vi "Autonomous Independent.vi"() -> ()   [LabVIEW 2016]
doc: "This VI is called when autonomous begins, and will automatically be terminated when autonomous ends. You can carry out timed or sensor driven robot movement independently without needing to return to the caller."
uses:
  <vilib>/Rock Robotics/WPI/Solenoid/WPI_SolenoidValue.ctl
  <vilib>/Rock Robotics/WPI/SafetyOutput/WPI_SafetyOutputConfigMenu.ctl
  <vilib>/Rock Robotics/WPI/Utilities/WPI_GetSetVariantRefNum.vi
  <vilib>/Rock Robotics/Network Tables/NT Read String.vi
  <vilib>/Rock Robotics/Network Tables/NT Write Numeric Array.vi
  <vilib>/Rock Robotics/WPI/Ultrasonic/WPI_SonarMB1010AnalogRefNum Registry Get.vi
  <vilib>/Rock Robotics/WPI/RobotDrive/WPI_RobotDriveArcadeDrive_Standard(NoSaturation).vi
  <vilib>/Rock Robotics/WPI/Solenoid/WPI_SolenoidSetEnum.vi
  <vilib>/addons/control/pid/pid.llb/PID (DBL).vi
  <vilib>/Rock Robotics/WPI/Ultrasonic/WPI_SonarMB1010AnalogGetRange.vi
  <vilib>/Rock Robotics/WPI/ThirdParty/Sensors/ADIS16448 IMU/ADIS16448_IMU.lvlib
  <vilib>/addons/control/pid/NI_PID_pid.lvlib
panel:
  out "Current Movement, for debugging":T1 {"Y Joystick Value" scale=1.0..-1.0; "X Joystick Value" scale=-1.0..1.0}
  in  "Array of robot movements":T2(array[cluster])=[{"X Joystick Value"=0.39393939393939403, "Y Joystick Value"=0.0, "Delay (sec)"=1.0, "Movement Name"="turn"}, {"X Joystick Value"=-0.3737373737373737, "Y Joystick Value"=0.0, "Delay (sec)"=1.0, "Movement Name"="turn back"}] {"Y Joystick Value" scale=1.0..-1.0; "X Joystick Value" scale=-1.0..1.0}
  # "Be sure to right-click and choose Data Operations>>Make Current Value default if you want to save the array values with the VI"
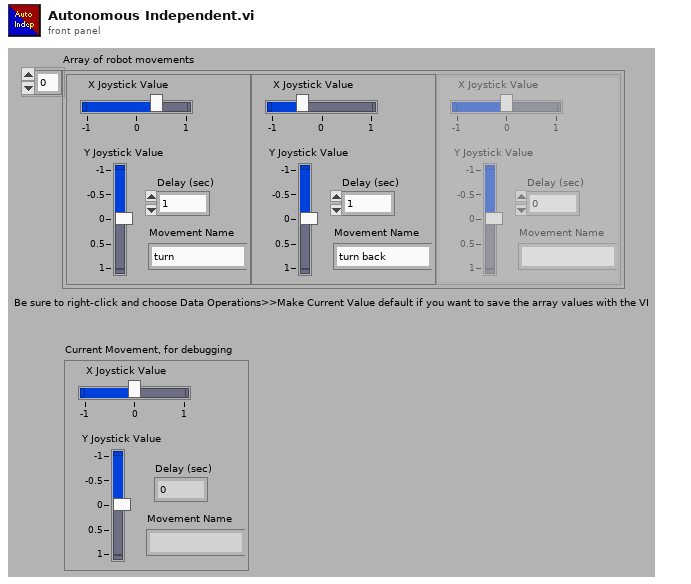
[diagram p1: front panel]
types:
  T1 = cluster{"X Joystick Value":dbl, "Y Joystick Value":dbl, "Delay (sec)":dbl, "Movement Name":string}
  T2 = cluster{"X Joystick Value":dbl, "Y Joystick Value":dbl, "Delay (sec)":dbl, "Movement Name":string}[]
  T3 = typedef "WPI_JoystickDevRef.ctl" = cluster{"Device":T4}
  T4 = typedef "WPI_JoystickDeviceEnum.ctl" = enum16{"USB 0", "USB 1", "USB 2", "USB 3", "USB 4", "USB 5"}
  T5 = typedef "WPI_RobotDriveDevRef.ctl" = cluster{"DevStatus":errorcluster, "Motors[]":T6[], "Square Inputs":bool, "Max Output":dbl}
  T6 = typedef "WPI_MotorControlDeviceRef.ctl" = cluster{"DeviceStatus":errorcluster, "Type":T7, "PWM":cluster{"PWM Channel":T8, "DeadBand":T9}, "CAN":cluster{"Device Number":u8, "SetOutput VI Ref":variant, "GetOutput VI Ref":variant, "Enable VI Ref":variant, "Disable VI Ref":variant, "Data":variant}, "Invert":bool}
  T7 = typedef "WPI_MotorControlType.ctl" = enum16{"PWM", "CAN"}
  T8 = typedef "FPGA_DIOPWMChannel.ctl" = enum8{"PWM 0", "PWM 1", "PWM 2", "PWM 3", "PWM 4", "PWM 5", "PWM 6", "PWM 7", "PWM 8", "PWM 9", "PWM MXP 0", "PWM MXP 1", "PWM MXP 2", "PWM MXP 3", "PWM MXP 4", "PWM MXP 5", "PWM MXP 6", "PWM MXP 7", "PWM MXP 8", "PWM MXP 9", "Invalid"}
  T9 = typedef "WPI_PWMDeadband.ctl" = cluster{"Name":string, "maxPositivePwm":i32, "minPositivePwm":i32, "centerPwm":i32, "maxNegativePwm":i32, "minNegativePwm":i32, "angularRange":u16}
  T10 = typedef "WPI_SonarMB1010AnalogDeviceRef.ctl" = cluster{"AIDeviceRef":T11, "Scaling factor (V/in)":dbl, "Average Bits":u8}
  T11 = typedef "WPI_AnalogChannelDevRef.ctl" = cluster{"DevStatus":errorcluster, "Analog Channel":T12}
  T12 = typedef "FPGA_AIChannel.ctl" = enum8{"AI 0", "AI 1", "AI 2", "AI 3", "AI MXP 0", "AI MXP 1", "AI MXP 2", "AI MXP 3", "Invalid"}
  T13 = typedef "WPI_SolenoidDevRef.ctl" = cluster{"DevStatus":errorcluster, "Pneumatics Control Module":u8, "Forward Solenoid Channel":T14, "Reverse Solenoid Channel":T14}
  T14 = typedef "WPI_SolenoidChannel.ctl" = enum8{"Solenoid 0", "Solenoid 1", "Solenoid 2", "Solenoid 3", "Solenoid 4", "Solenoid 5", "Solenoid 6", "Solenoid 7", "Invalid"}
  T15 = typedef "ADIS16448_IMU.lvlib/ADI_IMU_ADIS16448_InterruptDevRef.ctl" = cluster{"ADI IMU DevRef":T16, "InterruptRef":T18}
  T16 = typedef "ADIS16448_IMU.lvlib/ADI_IMU_ADIS16448_IMUDevRef.ctl" = cluster{"DevStatus":errorcluster, "Handle":i32, "SPI Bus":T17, "Device Found":bool, "Device Ready":bool, "Yaw Axis":enum16{"X", "Y", "Z"}, "AHRS Algorithm":enum16{"Complementary", "Madgwick"}, "Serial":u16, "Lot ID 2":u16, "Lot ID 1":u16, "Product ID":u16}
  T17 = typedef "spi_bus.ctl" = enum16{"SPI On-Board, CS0", "SPI On-Board, CS1", "SPI On-Board, CS2", "SPI On-Board, CS3", "SPI MXP", "Invalid"}
  T18 = typedef "WPI_InterruptRef.ctl" = cluster{"DevStatus":errorcluster, "InterruptIndex":T19}
  T19 = typedef "FPGA_InterruptIndex.ctl" = enum8{"0", "1", "2", "3", "4", "5", "6", "7", "Invalid"}
  T20 = typedef "WPI_SolenoidValue.ctl" = enum16{"Off", "On", "Forward", "Reverse"}
  T21 = typedef "WPI_SafetyOutputConfigMenu.ctl" = enum16{"Enable", "Disable"}
  T22 = cluster{"proportional gain (Kc)":dbl, "integral time (Ti, min)":dbl, "derivative time (Td, min)":dbl}
  T23 = cluster{"X Angle":dbl, "Y Angle":dbl, "Z Angle":dbl}
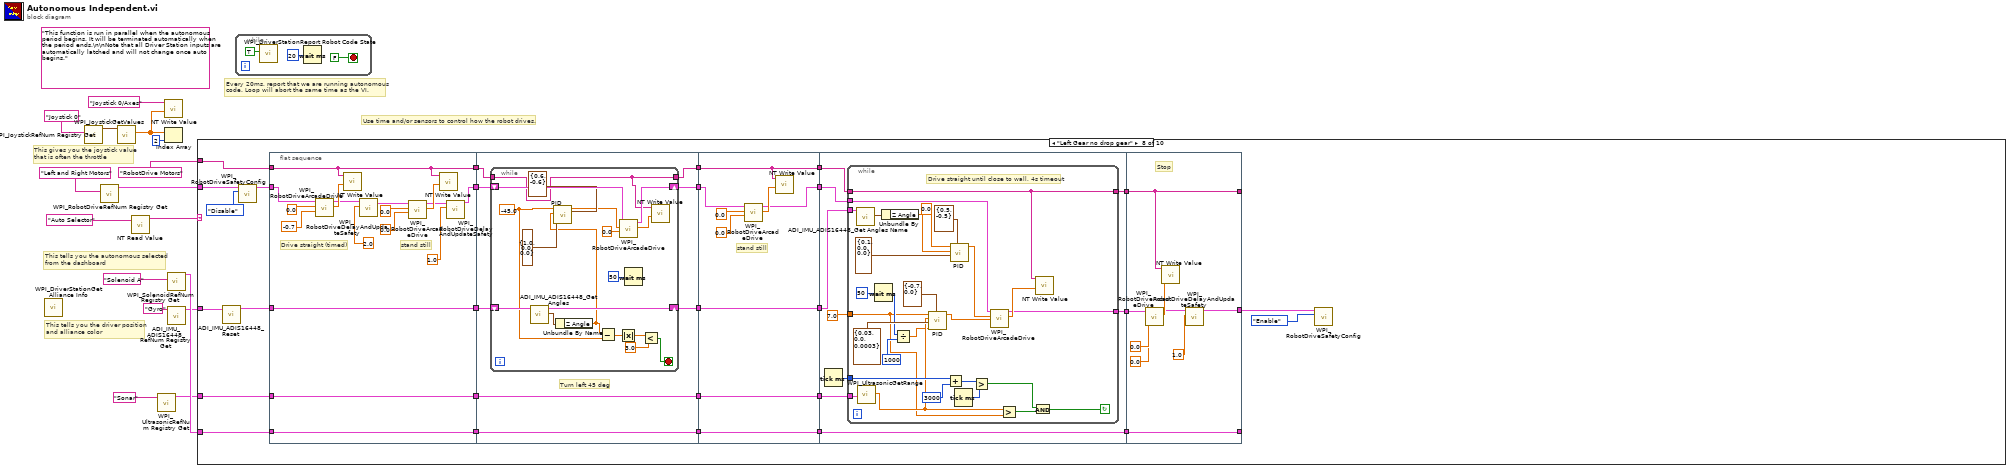
[diagram p0: block diagram]
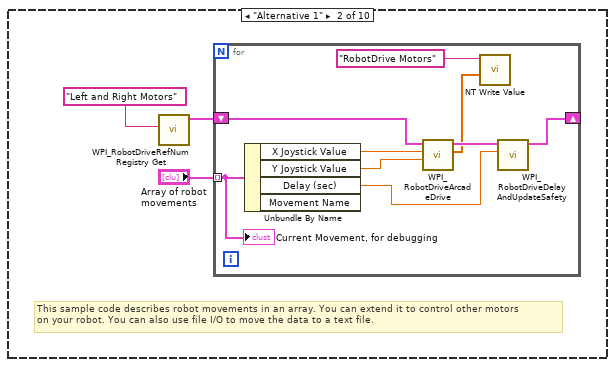
[diagram p3: hidden frame]
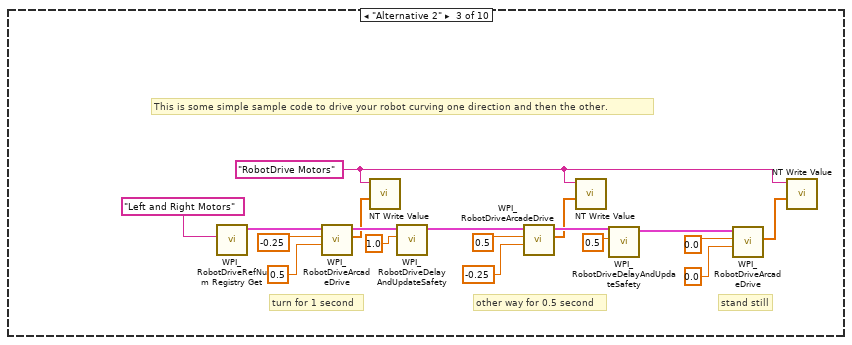
[diagram p4: hidden frame]
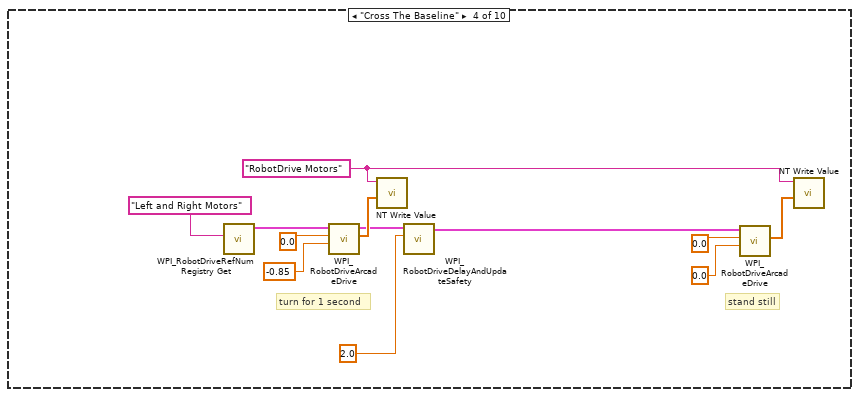
[diagram p5: hidden frame]
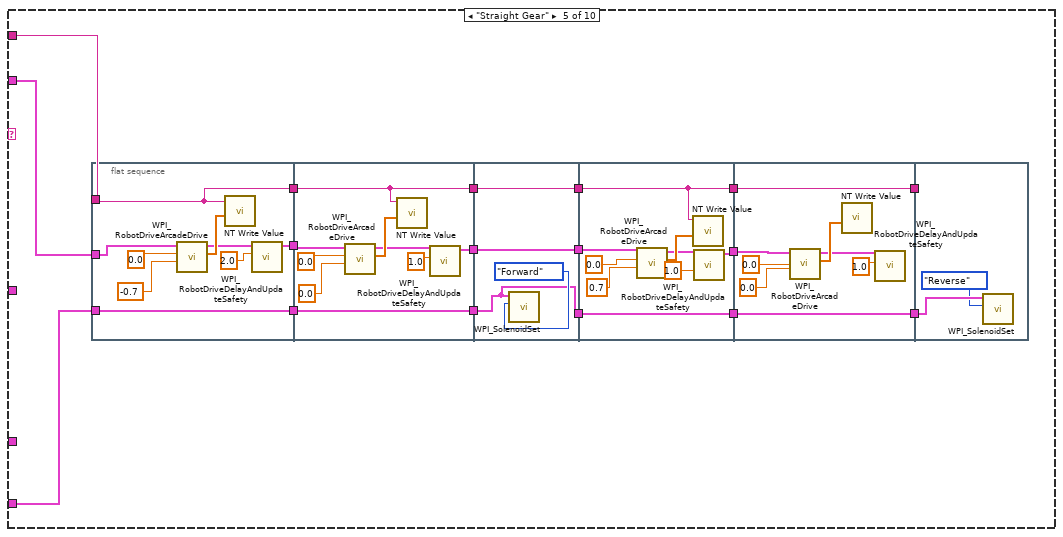
[diagram p6: hidden frame]
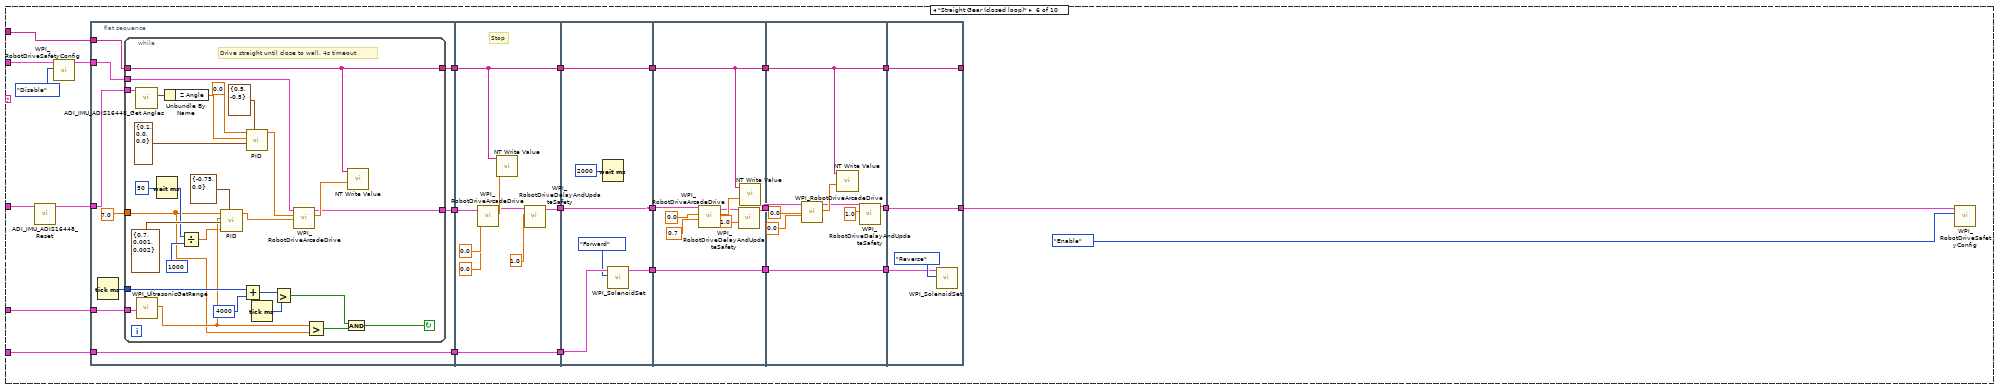
[diagram p7: hidden frame]
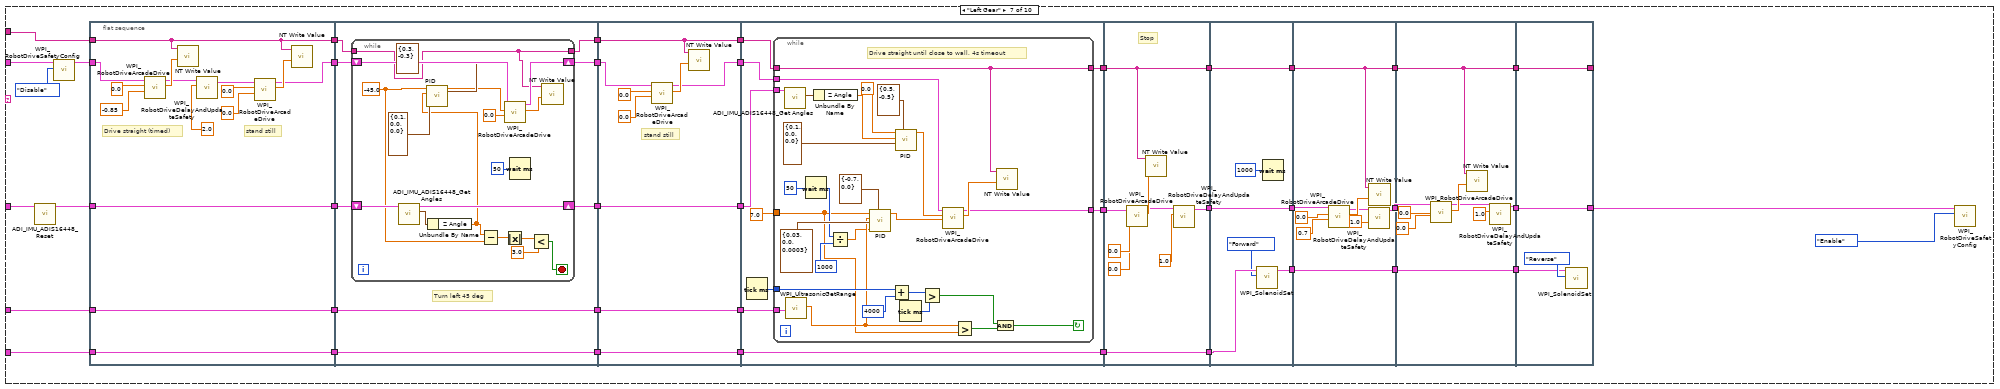
[diagram p8: hidden frame]
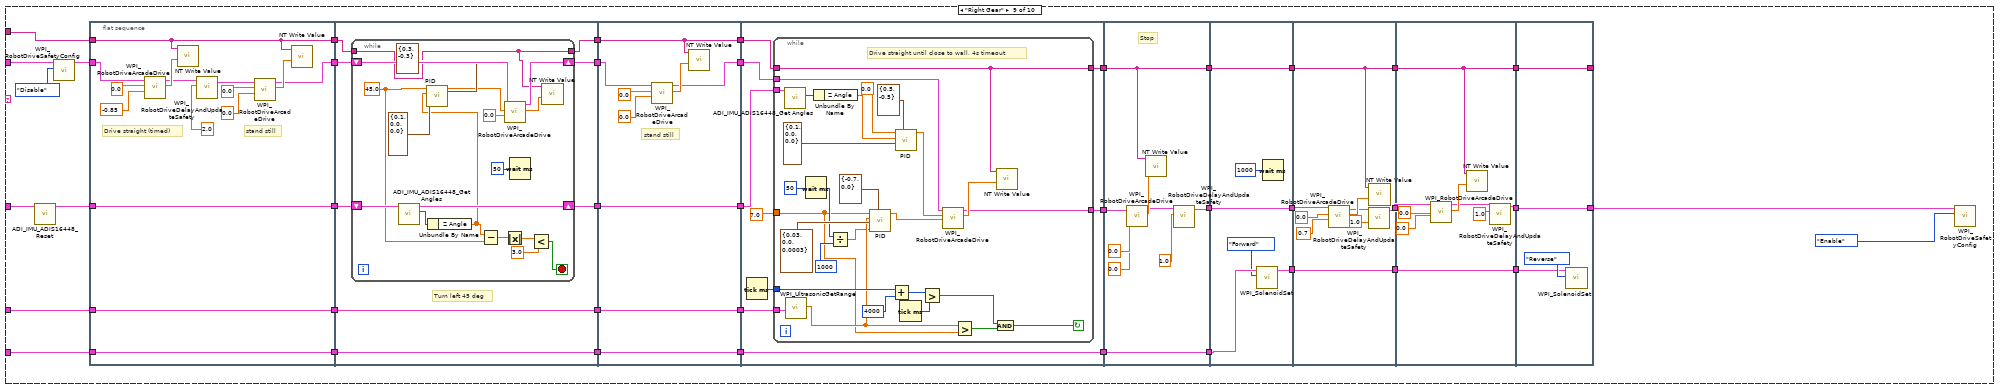
[diagram p9: hidden frame]
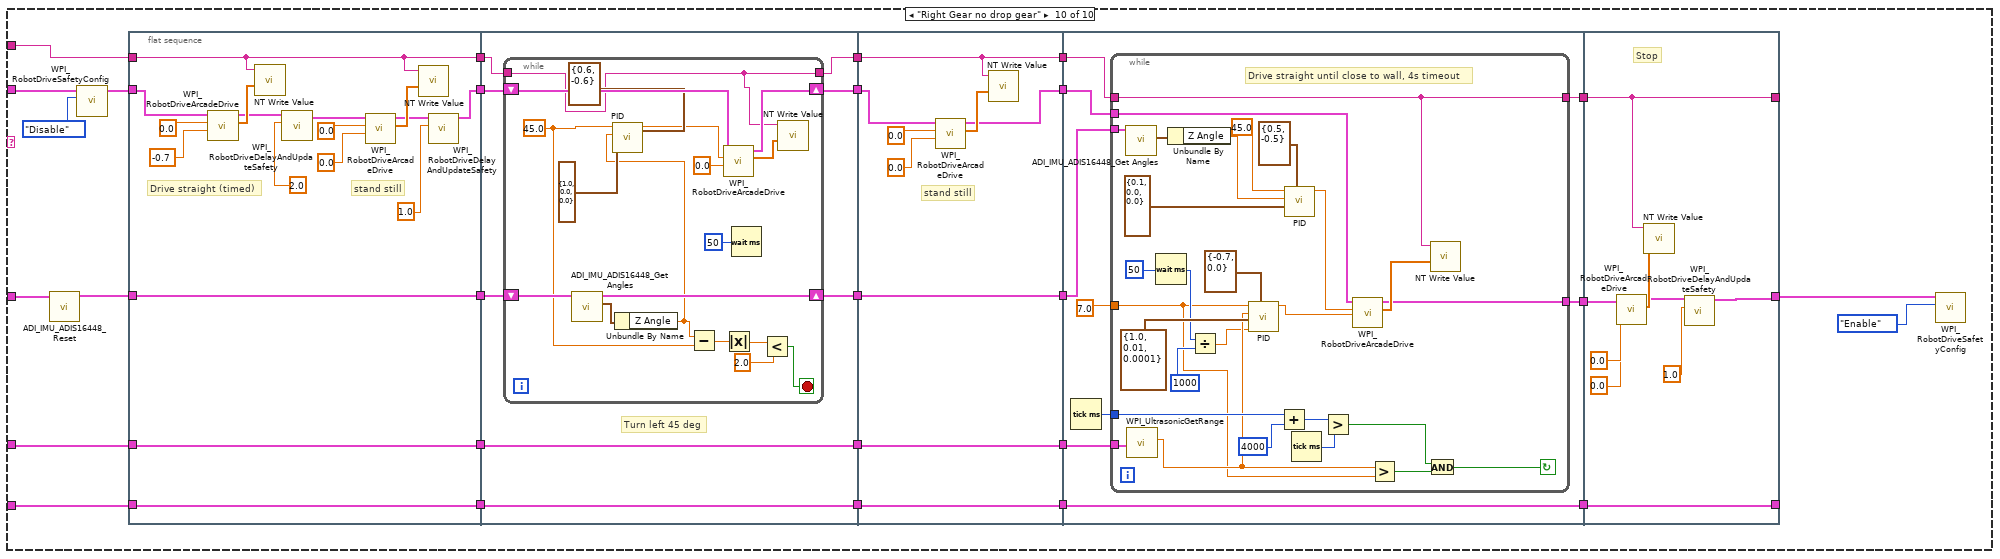
[diagram p10: hidden frame]
diagram:
  (unwired) "This function is run in parallel when the autonomous period begins. It will be terminated automatically when the period ends.\n\nNote that all Driver Station inputs are automatically latched and will not change once auto begins."
  # "This tells you the autonomous selected\nfrom the dashboard"
  # "Every 20ms, report that we are running autonomous\ncode. Loop will abort the same time as the VI."
  # "This gives you the joystick value\nthat is often the throttle"
  # "Use time and/or sensors to control how the robot drives."
  # "This tells you the driver position\nand alliance color"
  n1 = call <vilib>:"WPI_DriverStationGet Alliance Info.vi"() -> ()  [unwired: 12 out]
  n2 = call <vilib>:"WPI_JoystickRefNum Registry Get.vi"("refnum name"="Joystick 0") -> ("JoystickDevRef"=w15:T3)  [unwired: 1 in, 9 out]
  n3 = call <vilib>:"WPI_RobotDriveRefNum Registry Get.vi"("refnum name"="Left and Right Motors") -> ("RobotDriveDevRef"=w8:T5)  [unwired: 1 in, 9 out]
  n4 = call <vilib>:"WPI_JoystickGetValues.vi"("JoystickDevRef"=w15) -> ("Axes"=w11:dbl[])  [unwired: 6 in, 4 out]
  n5 = call-poly <vilib>:"NT Read Value.vi"("Name"="Auto Selector") -> ("String"=w12:string)  [unwired: 9 in, 1 out]
  n6 = call-poly <vilib>:"WPI_UltrasonicRefNum Registry Get.vi"("refnum name"="Sonar") -> ("SonarMB1010AnalogDevRef"=w1:T10)  [unwired: 9 in, 1 out]
  n7 = call-poly <vilib>:"NT Write Value.vi"("Numeric Array"=w11, "Name"="Joystick 0/Axes") -> ()  [unwired: 9 in, 1 out]
  n8 = Index Array(array=w11, index=2) -> ()  [unwired: 1 out]
  n9 = call <vilib>:"WPI_SolenoidRefNum Registry Get.vi"("refnum name"="Solenoid A") -> ("SolenoidDevRef"=w5:T13)  [unwired: 9 in, 1 out]
  n10 = call <vilib>:"ADI_IMU_ADIS16448_RefNum Registry Get.vi"("refnum name"="Gyro") -> ("ADI IMU Interrupt DevRef"=w3:T15)  [unwired: 9 in, 1 out]
  n11 = case shown="\"Left Gear no drop gear\"" w12 {
    tunnel: w8 -> [_ _ _ _ w75 w136 w249 w400 w537 w688]
    tunnel: "RobotDrive Motors" ("Name") -> [_ _ _ _ w74 w138 w251 w402 w539 w690]
    tunnel: w5 -> [_ _ _ _ w69 w137 w250 w401 w538 w689]
    tunnel: w3 -> [_ _ _ _ _ w141 w254 w405 w542 w693]
    tunnel: w1 -> [_ _ _ _ _ w140 w253 w404 w541 w692]
    frame Default {
      # "You can put your main auto here, or you can right-click on the case and make any\nother frame be the default case."
      # "This is the frame that will execute if no selection is made, or if it is not recognized"
    }
    frame "Alternative 1" {
      # "This sample code describes robot movements in an array. You can extend it to control other motors\non your robot. You can also use file I/O to move the data to a text file."
      n12 = call <vilib>:"WPI_RobotDriveRefNum Registry Get.vi"("refnum name"="Left and Right Motors") -> ("RobotDriveDevRef"=w18:T5)  [unwired: 1 in, 9 out]
      n13 = for {
        shift-right: [w26] -> _
        shift-left: w18 -> [w27]
        tunnel: "Array of robot movements" -> [w22] mode=indexing
        n14 = Unbundle By Name(w22) -> ("X Joystick Value"=w25:dbl, "Y Joystick Value"=w24:dbl, "Delay (sec)"=w23:dbl)  [unwired: 1 out]
        n15 = call-poly <vilib>:"WPI_RobotDriveArcadeDrive.vi"("Y axis value"=w24, "X axis value"=w25, "RobotDriveDevRef"=w27) -> ("Motor Values"=w20:dbl[], "RobotDriveDevRef"=w28:T5)  [unwired: 1 in, 6 out]
        n16 = call-poly <vilib>:"NT Write Value.vi"("Numeric Array"=w20, "Name"="RobotDrive Motors") -> ()  [unwired: 9 in, 1 out]
        n17 = call <vilib>:"WPI_RobotDriveDelayAndUpdateSafety.vi"("Delay (s)"=w23, "RobotDriveDevRef"=w28) -> ("RobotDriveDevRef 2"=w26:T5)  [unwired: 8 in, 1 out]
        "Current Movement, for debugging" <- w22
      }
    }
    frame "Alternative 2" {
      w30 = "RobotDrive Motors" ("Name")
      # "This is some simple sample code to drive your robot curving one direction and then the other."
      # "stand still"
      # "other way for 0.5 second"
      # "turn for 1 second"
      n18 = call <vilib>:"WPI_RobotDriveRefNum Registry Get.vi"("refnum name"="Left and Right Motors") -> ("RobotDriveDevRef"=w46:T5)  [unwired: 1 in, 9 out]
      n19 = call-poly <vilib>:"WPI_RobotDriveArcadeDrive.vi"("Y axis value"=0.5 ("X axis value"), "X axis value"=-0.25, "RobotDriveDevRef"=w46) -> ("Motor Values"=w29:dbl[], "RobotDriveDevRef"=w39:T5)  [unwired: 1 in, 6 out]
      n20 = call-poly <vilib>:"NT Write Value.vi"("Numeric Array"=w29, "Name"=w30) -> ()  [unwired: 9 in, 1 out]
      n21 = call <vilib>:"WPI_RobotDriveDelayAndUpdateSafety.vi"("Delay (s)"=1.0, "RobotDriveDevRef"=w39) -> ("RobotDriveDevRef 2"=w40:T5)  [unwired: 8 in, 1 out]
      n22 = call-poly <vilib>:"WPI_RobotDriveArcadeDrive.vi"("Y axis value"=-0.25 ("X axis value"), "X axis value"=0.5, "RobotDriveDevRef"=w40) -> ("Motor Values"=w31:dbl[], "RobotDriveDevRef"=w41:T5)  [unwired: 1 in, 6 out]
      n23 = call-poly <vilib>:"NT Write Value.vi"("Numeric Array"=w31, "Name"=w30) -> ()  [unwired: 9 in, 1 out]
      n24 = call <vilib>:"WPI_RobotDriveDelayAndUpdateSafety.vi"("Delay (s)"=0.5, "RobotDriveDevRef"=w41) -> ("RobotDriveDevRef 2"=w42:T5)  [unwired: 8 in, 1 out]
      n25 = call-poly <vilib>:"WPI_RobotDriveArcadeDrive.vi"("Y axis value"=0.0 ("X axis value"), "X axis value"=0.0, "RobotDriveDevRef"=w42) -> ("Motor Values"=w32:dbl[])  [unwired: 1 in, 7 out]
      n26 = call-poly <vilib>:"NT Write Value.vi"("Numeric Array"=w32, "Name"=w30) -> ()  [unwired: 9 in, 1 out]
    }
    frame "Cross The Baseline" {
      w57 = "RobotDrive Motors" ("Name")
      # "stand still"
      # "turn for 1 second"
      n27 = call <vilib>:"WPI_RobotDriveRefNum Registry Get.vi"("refnum name"="Left and Right Motors") -> ("RobotDriveDevRef"=w48:T5)  [unwired: 1 in, 9 out]
      n28 = call-poly <vilib>:"WPI_RobotDriveArcadeDrive.vi"("Y axis value"=-0.85 ("X axis value"), "X axis value"=0.0, "RobotDriveDevRef"=w48) -> ("Motor Values"=w58:dbl[], "RobotDriveDevRef"=w51:T5)  [unwired: 1 in, 6 out]
      n29 = call-poly <vilib>:"NT Write Value.vi"("Numeric Array"=w58, "Name"=w57) -> ()  [unwired: 9 in, 1 out]
      n30 = call <vilib>:"WPI_RobotDriveDelayAndUpdateSafety.vi"("Delay (s)"=2.0, "RobotDriveDevRef"=w51) -> ("RobotDriveDevRef 2"=w47:T5)  [unwired: 8 in, 1 out]
      n31 = call-poly <vilib>:"WPI_RobotDriveArcadeDrive.vi"("Y axis value"=0.0 ("X axis value"), "X axis value"=0.0, "RobotDriveDevRef"=w47) -> ("Motor Values"=w56:dbl[])  [unwired: 1 in, 7 out]
      n32 = call-poly <vilib>:"NT Write Value.vi"("Numeric Array"=w56, "Name"=w57) -> ()  [unwired: 9 in, 1 out]
    }
    frame "Straight Gear" {
      n33 = flat-sequence {
        tunnel: w75 -> [w79]
        tunnel: w74 -> [w77]
        tunnel: [w78] -> w73
        tunnel: [w77] -> w72
        tunnel: w69 -> [w76]
        tunnel: [w76] -> w68
        tunnel: w73 -> [w88]
        tunnel: w72 -> [w87]
        tunnel: [w87] -> w71
        tunnel: w68 -> [w86]
        tunnel: [w86] -> w67
        tunnel: [w85] -> w64
        tunnel: w71 -> [w97]
        tunnel: [w97] -> w70
        tunnel: w67 -> [w94]
        tunnel: w64 -> [w95]
        tunnel: [w95] -> w63
        tunnel: [w94] -> w61
        tunnel: w70 -> [w103]
        tunnel: [w103] -> w66
        tunnel: w63 -> [w102]
        tunnel: [w99] -> w62
        tunnel: w61 -> [w101]
        tunnel: [w101] -> w60
        tunnel: w66 -> [w114]
        tunnel: [w114] -> w65
        tunnel: w62 -> [w108]
        tunnel: w60 -> [w107]
        tunnel: [w107] -> w59
        tunnel: w65 -> [_]
        tunnel: w59 -> [w116]
        frame #0 {
          n34 = call-poly <vilib>:"WPI_RobotDriveArcadeDrive.vi"("Y axis value"=-0.7 ("X axis value"), "X axis value"=0.0, "RobotDriveDevRef"=w79) -> ("Motor Values"=w84:dbl[], "RobotDriveDevRef"=w81:T5)  [unwired: 1 in, 6 out]
          n35 = call-poly <vilib>:"NT Write Value.vi"("Numeric Array"=w84, "Name"=w77) -> ()  [unwired: 9 in, 1 out]
          n36 = call <vilib>:"WPI_RobotDriveDelayAndUpdateSafety.vi"("Delay (s)"=2.0, "RobotDriveDevRef"=w81) -> ("RobotDriveDevRef 2"=w78:T5)  [unwired: 8 in, 1 out]
        }
        frame #1 {
          n37 = call-poly <vilib>:"WPI_RobotDriveArcadeDrive.vi"("Y axis value"=0.0 ("X axis value"), "X axis value"=0.0, "RobotDriveDevRef"=w88) -> ("Motor Values"=w93:dbl[], "RobotDriveDevRef"=w90:T5)  [unwired: 1 in, 6 out]
          n38 = call-poly <vilib>:"NT Write Value.vi"("Numeric Array"=w93, "Name"=w87) -> ()  [unwired: 9 in, 1 out]
          n39 = call <vilib>:"WPI_RobotDriveDelayAndUpdateSafety.vi"("Delay (s)"=1.0, "RobotDriveDevRef"=w90) -> ("RobotDriveDevRef 2"=w85:T5)  [unwired: 8 in, 1 out]
        }
        frame #2 {
          n40 = call-poly <vilib>:"WPI_SolenoidSet.vi"("Value"=WPI_SolenoidValue."Forward", "SolenoidDevRef"=w94) -> ()  [unwired: 8 in, 2 out]
        }
        frame #3 {
          w98 = 1.0 ("Delay (s)")
          n41 = call-poly <vilib>:"WPI_RobotDriveArcadeDrive.vi"("Y axis value"=0.7 ("X axis value"), "X axis value"=0.0, "RobotDriveDevRef"=w102) -> ("Motor Values"=w106:dbl[], "RobotDriveDevRef"=w100:T5)  [unwired: 1 in, 6 out]
          n42 = call-poly <vilib>:"NT Write Value.vi"("Numeric Array"=w106, "Name"=w103) -> ()  [unwired: 9 in, 1 out]
          n43 = call <vilib>:"WPI_RobotDriveDelayAndUpdateSafety.vi"("Feed time (s)"=w98, "Delay (s)"=w98, "RobotDriveDevRef"=w100) -> ("RobotDriveDevRef 2"=w99:T5)  [unwired: 7 in, 1 out]
        }
        frame #4 {
          n44 = call-poly <vilib>:"WPI_RobotDriveArcadeDrive.vi"("Y axis value"=0.0 ("X axis value"), "X axis value"=0.0, "RobotDriveDevRef"=w108) -> ("Motor Values"=w113:dbl[], "RobotDriveDevRef"=w111:T5)  [unwired: 1 in, 6 out]
          n45 = call-poly <vilib>:"NT Write Value.vi"("Numeric Array"=w113) -> ()  [unwired: 10 in, 1 out]
          n46 = call <vilib>:"WPI_RobotDriveDelayAndUpdateSafety.vi"("Delay (s)"=1.0, "RobotDriveDevRef"=w111) -> ()  [unwired: 8 in, 2 out]
        }
        frame #5 {
          n47 = call-poly <vilib>:"WPI_SolenoidSet.vi"("Value"=WPI_SolenoidValue."Reverse", "SolenoidDevRef"=w116) -> ()  [unwired: 8 in, 2 out]
        }
      }
    }
    frame "Straight Gear (closed loop)" {
      n48 = call <vilib>:"ADI_IMU_ADIS16448_Reset.vi"("ADI IMU Interrupt DevRef"=w141) -> ("ADI IMU Interrupt DevRef Out"=w139:T15)  [unwired: 9 in, 1 out]
      n49 = call <vilib>:"WPI_RobotDriveSafetyConfig.vi"("mode"=WPI_SafetyOutputConfigMenu."Disable", "RobotDriveDevRef"=w136) -> ("RobotDriveDevRef"=w135:T5)  [unwired: 8 in, 1 out]
      n50 = flat-sequence {
        tunnel: w140 -> [w150]
        tunnel: w139 -> [w143]
        tunnel: w138 -> [w148]
        tunnel: w135 -> [w147]
        tunnel: w137 -> [w142]
        tunnel: [w146] -> w131
        tunnel: [w145] -> w130
        tunnel: [w142] -> w127
        tunnel: w131 -> [w186]
        tunnel: w130 -> [w182]
        tunnel: [w179] -> w129
        tunnel: [w182] -> w128
        tunnel: w127 -> [w181]
        tunnel: [w181] -> w126
        tunnel: w129 -> [w188]
        tunnel: w128 -> [w192]
        tunnel: w126 -> [w191]
        tunnel: [w188] -> w125
        tunnel: [w192] -> w124
        tunnel: [w190] -> w123
        tunnel: w125 -> [w193]
        tunnel: w124 -> [w194]
        tunnel: w123 -> [w201]
        tunnel: [w195] -> w122
        tunnel: [w194] -> w121
        tunnel: [w201] -> w120
        tunnel: w122 -> [w204]
        tunnel: w121 -> [w202]
        tunnel: w120 -> [w210]
        tunnel: [w203] -> w119
        tunnel: [w202] -> w118
        tunnel: [w210] -> w117
        tunnel: [w213] -> _
        tunnel: [w214] -> w133
        tunnel: w119 -> [w214]
        tunnel: w118 -> [w213]
        tunnel: w117 -> [w211]
        frame #0 {
          n51 = Tick Count (ms)() -> (millisecond timer value=w149:u32)
          n52 = while {
            tunnel: w150 -> [w177]
            tunnel: w149 -> [w175]
            tunnel: w148 -> [w164]
            tunnel: w147 -> [w169]
            tunnel: [w168] -> w146
            tunnel: [w164] -> w145
            tunnel: 7.0 ("setpoint") -> [w159]
            tunnel: w143 -> [w158]
            stop <- w161 continue-if-true
            w167 = u32 50 ("milliseconds to wait")
            # "Drive straight until close to wall, 4s timeout"
            n53 = call <vilib>:"ADI_IMU_ADIS16448_Get Angles.vi"("ADI IMU Interrupt DevRef"=w158) -> ("IMU Angles Out"=w153:T23)  [unwired: 7 in, 3 out]
            n54 = call-poly <vilib>:"WPI_UltrasonicGetRange.vi"("SonarMB1010AnalogDevRef"=w177) -> ("Distance"=w171:dbl)  [unwired: 8 in, 2 out]
            n55 = Wait (ms)(milliseconds to wait=w167) -> ()  [unwired: 1 out]
            n56 = Unbundle By Name(w153) -> ("Z Angle"=w152:dbl)
            n57 = Divide(x=w167, y=u32 1000) -> (x/y=w165:dbl)
            n58 = call-poly <vilib>:"PID.vi"("output range"=cluster{"output high":dbl, "output low":dbl} {"output high"=-0.75, "output low"=0.0}, "dt (s)"=w165, "PID gains"=T22 {"proportional gain (Kc)"=0.7, "integral time (Ti, min)"=0.001, "derivative time (Td, min)"=0.002}, "process variable"=w171, "setpoint"=w159) -> ("output"=w151:dbl)  [unwired: 5 in, 1 out]
            n59 = Add(x=w175, y=u32 4000) -> (x+y=w163:u32)
            n60 = call-poly <vilib>:"PID.vi"("output range"=cluster{"output high":dbl, "output low":dbl} {"output high"=0.5, "output low"=-0.5}, "PID gains"=T22 {"proportional gain (Kc)"=0.1, "integral time (Ti, min)"=0.0, "derivative time (Td, min)"=0.0}, "process variable"=w152, "setpoint"=0.0) -> ("output"=w155:dbl)  [unwired: 6 in, 1 out]
            n61 = Tick Count (ms)() -> (millisecond timer value=w162:u32)
            n62 = Greater?(x=w163, y=w162) -> (0:w160:bool)
            n63 = call-poly <vilib>:"WPI_RobotDriveArcadeDrive.vi"("Y axis value"=w151, "X axis value"=w155, "RobotDriveDevRef"=w169) -> ("Motor Values"=w170:dbl[], "RobotDriveDevRef"=w168:T5)  [unwired: 6 in, 1 out]
            n64 = Greater?(x=w171, y=w159) -> (0:w176:bool)
            n65 = And(x=w160, y=w176) -> (x .and. y?=w161:bool)
            n66 = call-poly <vilib>:"NT Write Value.vi"("Numeric Array"=w170, "Name"=w164) -> ()  [unwired: 9 in, 1 out]
          }
        }
        frame #1 {
          # "Stop"
          n67 = call-poly <vilib>:"WPI_RobotDriveArcadeDrive.vi"("Y axis value"=0.0, "X axis value"=0.0, "RobotDriveDevRef"=w186) -> ("Motor Values"=w185:dbl[], "RobotDriveDevRef"=w180:T5)  [unwired: 6 in, 1 out]
          n68 = call-poly <vilib>:"NT Write Value.vi"("Numeric Array"=w185, "Name"=w182) -> ()  [unwired: 9 in, 1 out]
          n69 = call <vilib>:"WPI_RobotDriveDelayAndUpdateSafety.vi"("Delay (s)"=1.0, "RobotDriveDevRef"=w180) -> ("RobotDriveDevRef 2"=w179:T5)  [unwired: 8 in, 1 out]
        }
        frame #2 {
          n70 = Wait (ms)(milliseconds to wait=u32 2000) -> ()  [unwired: 1 out]
          n71 = call-poly <vilib>:"WPI_SolenoidSet.vi"("Value"=WPI_SolenoidValue."Forward", "SolenoidDevRef"=w191) -> ("SolenoidDevRef"=w190:T13)  [unwired: 8 in, 1 out]
        }
        frame #3 {
          n72 = call-poly <vilib>:"WPI_RobotDriveArcadeDrive.vi"("Y axis value"=0.7 ("X axis value"), "X axis value"=0.0, "RobotDriveDevRef"=w193) -> ("Motor Values"=w200:dbl[], "RobotDriveDevRef"=w197:T5)  [unwired: 1 in, 6 out]
          n73 = call <vilib>:"WPI_RobotDriveDelayAndUpdateSafety.vi"("Delay (s)"=1.0, "RobotDriveDevRef"=w197) -> ("RobotDriveDevRef 2"=w195:T5)  [unwired: 8 in, 1 out]
          n74 = call-poly <vilib>:"NT Write Value.vi"("Numeric Array"=w200, "Name"=w194) -> ()  [unwired: 9 in, 1 out]
        }
        frame #4 {
          n75 = call-poly <vilib>:"WPI_RobotDriveArcadeDrive.vi"("Y axis value"=0.0 ("X axis value"), "X axis value"=0.0, "RobotDriveDevRef"=w204) -> ("Motor Values"=w209:dbl[], "RobotDriveDevRef"=w207:T5)  [unwired: 1 in, 6 out]
          n76 = call-poly <vilib>:"NT Write Value.vi"("Numeric Array"=w209, "Name"=w202) -> ()  [unwired: 9 in, 1 out]
          n77 = call <vilib>:"WPI_RobotDriveDelayAndUpdateSafety.vi"("Delay (s)"=1.0, "RobotDriveDevRef"=w207) -> ("RobotDriveDevRef 2"=w203:T5)  [unwired: 8 in, 1 out]
        }
        frame #5 {
          n78 = call-poly <vilib>:"WPI_SolenoidSet.vi"("Value"=WPI_SolenoidValue."Reverse", "SolenoidDevRef"=w211) -> ()  [unwired: 8 in, 2 out]
        }
      }
      n79 = call <vilib>:"WPI_RobotDriveSafetyConfig.vi"("mode"=WPI_SafetyOutputConfigMenu."Enable", "RobotDriveDevRef"=w133) -> ()  [unwired: 8 in, 2 out]
    }
    frame "Left Gear" {
      n80 = call <vilib>:"ADI_IMU_ADIS16448_Reset.vi"("ADI IMU Interrupt DevRef"=w254) -> ("ADI IMU Interrupt DevRef Out"=w252:T15)  [unwired: 9 in, 1 out]
      n81 = call <vilib>:"WPI_RobotDriveSafetyConfig.vi"("mode"=WPI_SafetyOutputConfigMenu."Disable", "RobotDriveDevRef"=w249) -> ("RobotDriveDevRef"=w248:T5)  [unwired: 8 in, 1 out]
      n82 = flat-sequence {
        tunnel: w250 -> [w267]
        tunnel: w248 -> [w257]
        tunnel: w251 -> [w256]
        tunnel: w252 -> [w268]
        tunnel: w253 -> [w269]
        tunnel: [w269] -> w219
        tunnel: [w268] -> w218
        tunnel: [w256] -> w217
        tunnel: [w255] -> w216
        tunnel: [w267] -> w215
        tunnel: [w277] -> w224
        tunnel: [w272] -> w223
        tunnel: [w270] -> w222
        tunnel: [w274] -> w221
        tunnel: [w276] -> w220
        tunnel: w219 -> [w277]
        tunnel: w218 -> [w273]
        tunnel: w217 -> [w271]
        tunnel: w216 -> [w275]
        tunnel: w215 -> [w276]
        tunnel: [w304] -> w229
        tunnel: [w303] -> w228
        tunnel: [w298] -> w227
        tunnel: [w296] -> w226
        tunnel: [w302] -> w225
        tunnel: w224 -> [w304]
        tunnel: w223 -> [w303]
        tunnel: w222 -> [w298]
        tunnel: w221 -> [w297]
        tunnel: w220 -> [w302]
        tunnel: [w309] -> w244
        tunnel: [w308] -> w243
        tunnel: [w305] -> w240
        tunnel: w229 -> [w313]
        tunnel: w228 -> [w306]
        tunnel: w227 -> [w311]
        tunnel: w226 -> [w310]
        tunnel: w225 -> [w305]
        tunnel: w244 -> [w349]
        tunnel: w243 -> [w345]
        tunnel: [w342] -> w242
        tunnel: [w345] -> w241
        tunnel: w240 -> [w344]
        tunnel: [w344] -> w239
        tunnel: w242 -> [w355]
        tunnel: w241 -> [w354]
        tunnel: w239 -> [w353]
        tunnel: [w355] -> w238
        tunnel: [w354] -> w237
        tunnel: [w352] -> w236
        tunnel: w238 -> [w358]
        tunnel: w237 -> [w356]
        tunnel: w236 -> [w364]
        tunnel: [w357] -> w235
        tunnel: [w356] -> w234
        tunnel: [w364] -> w233
        tunnel: w235 -> [w367]
        tunnel: w234 -> [w365]
        tunnel: w233 -> [w373]
        tunnel: [w366] -> w232
        tunnel: [w365] -> w231
        tunnel: [w373] -> w230
        tunnel: [w376] -> _
        tunnel: [w377] -> w246
        tunnel: w232 -> [w377]
        tunnel: w231 -> [w376]
        tunnel: w230 -> [w374]
        frame #0 {
          # "stand still"
          # "Drive straight (timed)"
          n83 = call-poly <vilib>:"WPI_RobotDriveArcadeDrive.vi"("Y axis value"=-0.85 ("X axis value"), "X axis value"=0.0, "RobotDriveDevRef"=w257) -> ("Motor Values"=w266:dbl[], "RobotDriveDevRef"=w260:T5)  [unwired: 1 in, 6 out]
          n84 = call-poly <vilib>:"NT Write Value.vi"("Numeric Array"=w266, "Name"=w256) -> ()  [unwired: 9 in, 1 out]
          n85 = call <vilib>:"WPI_RobotDriveDelayAndUpdateSafety.vi"("Delay (s)"=2.0, "RobotDriveDevRef"=w260) -> ("RobotDriveDevRef 2"=w258:T5)  [unwired: 8 in, 1 out]
          n86 = call-poly <vilib>:"WPI_RobotDriveArcadeDrive.vi"("Y axis value"=0.0 ("X axis value"), "X axis value"=0.0, "RobotDriveDevRef"=w258) -> ("Motor Values"=w265:dbl[], "RobotDriveDevRef"=w255:T5)  [unwired: 1 in, 6 out]
          n87 = call-poly <vilib>:"NT Write Value.vi"("Numeric Array"=w265, "Name"=w256) -> ()  [unwired: 9 in, 1 out]
        }
        frame #1 {
          # "Turn left 45 deg"
          n88 = while {
            shift-right: [w293] -> w274
            shift-left: w275 -> [w294]
            shift-right: [w290] -> w272
            shift-left: w273 -> [w291]
            tunnel: w271 -> [w284]
            tunnel: [w284] -> w270
            stop <- w278 stop-if-true
            w282 = -45.0 ("setpoint")
            n89 = call <vilib>:"ADI_IMU_ADIS16448_Get Angles.vi"("ADI IMU Interrupt DevRef"=w291) -> ("IMU Angles Out"=w292:T23, "ADI IMU Interrupt DevRef Out"=w290:T15)  [unwired: 7 in, 2 out]
            n90 = Unbundle By Name(w292) -> ("Z Angle"=w283:dbl)
            n91 = call-poly <vilib>:"PID.vi"("output range"=cluster{"output high":dbl, "output low":dbl} {"output high"=0.3, "output low"=-0.3}, "PID gains"=T22 {"proportional gain (Kc)"=0.1, "integral time (Ti, min)"=0.0, "derivative time (Td, min)"=0.0}, "process variable"=w283, "setpoint"=w282) -> ("output"=w287:dbl)  [unwired: 6 in, 1 out]
            n92 = Subtract(x=w283, y=w282) -> (x-y=w281:dbl)
            n93 = call-poly <vilib>:"WPI_RobotDriveArcadeDrive.vi"("Y axis value"=0.0, "X axis value"=w287, "RobotDriveDevRef"=w294) -> ("Motor Values"=w285:dbl[], "RobotDriveDevRef"=w293:T5)  [unwired: 6 in, 1 out]
            n94 = Absolute Value(x=w281) -> (abs(x)=w280:dbl)
            n95 = Wait (ms)(milliseconds to wait=u32 50) -> ()  [unwired: 1 out]
            n96 = Less?(x=w280, y=3.0) -> (x < y?=w278:bool)
            n97 = call-poly <vilib>:"NT Write Value.vi"("Numeric Array"=w285, "Name"=w284) -> ()  [unwired: 9 in, 1 out]
          }
        }
        frame #2 {
          # "stand still"
          n98 = call-poly <vilib>:"WPI_RobotDriveArcadeDrive.vi"("Y axis value"=0.0 ("X axis value"), "X axis value"=0.0, "RobotDriveDevRef"=w297) -> ("Motor Values"=w301:dbl[], "RobotDriveDevRef"=w296:T5)  [unwired: 1 in, 6 out]
          n99 = call-poly <vilib>:"NT Write Value.vi"("Numeric Array"=w301, "Name"=w298) -> ()  [unwired: 9 in, 1 out]
        }
        frame #3 {
          n100 = Tick Count (ms)() -> (millisecond timer value=w312:u32)
          n101 = while {
            tunnel: w313 -> [w340]
            tunnel: w312 -> [w338]
            tunnel: w311 -> [w327]
            tunnel: w310 -> [w332]
            tunnel: [w331] -> w309
            tunnel: [w327] -> w308
            tunnel: 7.0 ("setpoint") -> [w322]
            tunnel: w306 -> [w321]
            stop <- w324 continue-if-true
            w330 = u32 50 ("milliseconds to wait")
            # "Drive straight until close to wall, 4s timeout"
            n102 = call <vilib>:"ADI_IMU_ADIS16448_Get Angles.vi"("ADI IMU Interrupt DevRef"=w321) -> ("IMU Angles Out"=w316:T23)  [unwired: 7 in, 3 out]
            n103 = call-poly <vilib>:"WPI_UltrasonicGetRange.vi"("SonarMB1010AnalogDevRef"=w340) -> ("Distance"=w334:dbl)  [unwired: 8 in, 2 out]
            n104 = Wait (ms)(milliseconds to wait=w330) -> ()  [unwired: 1 out]
            n105 = Unbundle By Name(w316) -> ("Z Angle"=w315:dbl)
            n106 = Divide(x=w330, y=u32 1000) -> (x/y=w328:dbl)
            n107 = call-poly <vilib>:"PID.vi"("output range"=cluster{"output high":dbl, "output low":dbl} {"output high"=-0.7, "output low"=0.0}, "dt (s)"=w328, "PID gains"=T22 {"proportional gain (Kc)"=0.03, "integral time (Ti, min)"=0.0, "derivative time (Td, min)"=0.0003}, "process variable"=w334, "setpoint"=w322) -> ("output"=w314:dbl)  [unwired: 5 in, 1 out]
            n108 = Add(x=w338, y=u32 4000) -> (x+y=w326:u32)
            n109 = call-poly <vilib>:"PID.vi"("output range"=cluster{"output high":dbl, "output low":dbl} {"output high"=0.5, "output low"=-0.5}, "PID gains"=T22 {"proportional gain (Kc)"=0.1, "integral time (Ti, min)"=0.0, "derivative time (Td, min)"=0.0}, "process variable"=w315, "setpoint"=0.0) -> ("output"=w318:dbl)  [unwired: 6 in, 1 out]
            n110 = Tick Count (ms)() -> (millisecond timer value=w325:u32)
            n111 = Greater?(x=w326, y=w325) -> (0:w323:bool)
            n112 = call-poly <vilib>:"WPI_RobotDriveArcadeDrive.vi"("Y axis value"=w314, "X axis value"=w318, "RobotDriveDevRef"=w332) -> ("Motor Values"=w333:dbl[], "RobotDriveDevRef"=w331:T5)  [unwired: 6 in, 1 out]
            n113 = Greater?(x=w334, y=w322) -> (0:w339:bool)
            n114 = And(x=w323, y=w339) -> (x .and. y?=w324:bool)
            n115 = call-poly <vilib>:"NT Write Value.vi"("Numeric Array"=w333, "Name"=w327) -> ()  [unwired: 9 in, 1 out]
          }
        }
        frame #4 {
          # "Stop"
          n116 = call-poly <vilib>:"WPI_RobotDriveArcadeDrive.vi"("Y axis value"=0.0, "X axis value"=0.0, "RobotDriveDevRef"=w349) -> ("Motor Values"=w348:dbl[], "RobotDriveDevRef"=w343:T5)  [unwired: 6 in, 1 out]
          n117 = call-poly <vilib>:"NT Write Value.vi"("Numeric Array"=w348, "Name"=w345) -> ()  [unwired: 9 in, 1 out]
          n118 = call <vilib>:"WPI_RobotDriveDelayAndUpdateSafety.vi"("Delay (s)"=1.0, "RobotDriveDevRef"=w343) -> ("RobotDriveDevRef 2"=w342:T5)  [unwired: 8 in, 1 out]
        }
        frame #5 {
          n119 = call-poly <vilib>:"WPI_SolenoidSet.vi"("Value"=WPI_SolenoidValue."Forward", "SolenoidDevRef"=w353) -> ("SolenoidDevRef"=w352:T13)  [unwired: 8 in, 1 out]
          n120 = Wait (ms)(milliseconds to wait=u32 1000) -> ()  [unwired: 1 out]
        }
        frame #6 {
          n121 = call-poly <vilib>:"WPI_RobotDriveArcadeDrive.vi"("Y axis value"=0.7 ("X axis value"), "X axis value"=0.0, "RobotDriveDevRef"=w358) -> ("Motor Values"=w363:dbl[], "RobotDriveDevRef"=w360:T5)  [unwired: 1 in, 6 out]
          n122 = call <vilib>:"WPI_RobotDriveDelayAndUpdateSafety.vi"("Delay (s)"=1.0, "RobotDriveDevRef"=w360) -> ("RobotDriveDevRef 2"=w357:T5)  [unwired: 8 in, 1 out]
          n123 = call-poly <vilib>:"NT Write Value.vi"("Numeric Array"=w363, "Name"=w356) -> ()  [unwired: 9 in, 1 out]
        }
        frame #7 {
          n124 = call-poly <vilib>:"WPI_RobotDriveArcadeDrive.vi"("Y axis value"=0.0 ("X axis value"), "X axis value"=0.0, "RobotDriveDevRef"=w367) -> ("Motor Values"=w372:dbl[], "RobotDriveDevRef"=w370:T5)  [unwired: 1 in, 6 out]
          n125 = call-poly <vilib>:"NT Write Value.vi"("Numeric Array"=w372, "Name"=w365) -> ()  [unwired: 9 in, 1 out]
          n126 = call <vilib>:"WPI_RobotDriveDelayAndUpdateSafety.vi"("Delay (s)"=1.0, "RobotDriveDevRef"=w370) -> ("RobotDriveDevRef 2"=w366:T5)  [unwired: 8 in, 1 out]
        }
        frame #8 {
          n127 = call-poly <vilib>:"WPI_SolenoidSet.vi"("Value"=WPI_SolenoidValue."Reverse", "SolenoidDevRef"=w374) -> ()  [unwired: 8 in, 2 out]
        }
      }
      n128 = call <vilib>:"WPI_RobotDriveSafetyConfig.vi"("mode"=WPI_SafetyOutputConfigMenu."Enable", "RobotDriveDevRef"=w246) -> ()  [unwired: 8 in, 2 out]
    }
    frame "Left Gear no drop gear" {
      n129 = call <vilib>:"ADI_IMU_ADIS16448_Reset.vi"("ADI IMU Interrupt DevRef"=w405) -> ("ADI IMU Interrupt DevRef Out"=w403:T15)  [unwired: 9 in, 1 out]
      n130 = call <vilib>:"WPI_RobotDriveSafetyConfig.vi"("mode"=WPI_SafetyOutputConfigMenu."Disable", "RobotDriveDevRef"=w400) -> ("RobotDriveDevRef"=w399:T5)  [unwired: 8 in, 1 out]
      n131 = flat-sequence {
        tunnel: w401 -> [w420]
        tunnel: w399 -> [w410]
        tunnel: w402 -> [w409]
        tunnel: w403 -> [w421]
        tunnel: w404 -> [w422]
        tunnel: [w422] -> w383
        tunnel: [w421] -> w382
        tunnel: [w409] -> w381
        tunnel: [w407] -> w380
        tunnel: [w420] -> w379
        tunnel: [w430] -> w388
        tunnel: [w425] -> w387
        tunnel: [w423] -> w386
        tunnel: [w427] -> w385
        tunnel: [w429] -> w384
        tunnel: w383 -> [w430]
        tunnel: w382 -> [w426]
        tunnel: w381 -> [w424]
        tunnel: w380 -> [w428]
        tunnel: w379 -> [w429]
        tunnel: [w457] -> w393
        tunnel: [w456] -> w392
        tunnel: [w451] -> w391
        tunnel: [w449] -> w390
        tunnel: [w455] -> w389
        tunnel: w388 -> [w457]
        tunnel: w387 -> [w456]
        tunnel: w386 -> [w451]
        tunnel: w385 -> [w450]
        tunnel: w384 -> [w455]
        tunnel: [w462] -> w396
        tunnel: [w461] -> w395
        tunnel: [w458] -> w394
        tunnel: w393 -> [w466]
        tunnel: w392 -> [w459]
        tunnel: w391 -> [w464]
        tunnel: w390 -> [w463]
        tunnel: w389 -> [w458]
        tunnel: [w502] -> w378
        tunnel: w394 -> [w495]
        tunnel: w395 -> [w494]
        tunnel: w396 -> [w501]
        tunnel: [w495] -> _
        tunnel: [w494] -> _
        frame #0 {
          # "stand still"
          # "Drive straight (timed)"
          n132 = call-poly <vilib>:"WPI_RobotDriveArcadeDrive.vi"("Y axis value"=-0.7 ("X axis value"), "X axis value"=0.0, "RobotDriveDevRef"=w410) -> ("Motor Values"=w419:dbl[], "RobotDriveDevRef"=w413:T5)  [unwired: 1 in, 6 out]
          n133 = call-poly <vilib>:"NT Write Value.vi"("Numeric Array"=w419, "Name"=w409) -> ()  [unwired: 9 in, 1 out]
          n134 = call <vilib>:"WPI_RobotDriveDelayAndUpdateSafety.vi"("Delay (s)"=2.0, "RobotDriveDevRef"=w413) -> ("RobotDriveDevRef 2"=w411:T5)  [unwired: 8 in, 1 out]
          n135 = call-poly <vilib>:"WPI_RobotDriveArcadeDrive.vi"("Y axis value"=0.0 ("X axis value"), "X axis value"=0.0, "RobotDriveDevRef"=w411) -> ("Motor Values"=w418:dbl[], "RobotDriveDevRef"=w408:T5)  [unwired: 1 in, 6 out]
          n136 = call-poly <vilib>:"NT Write Value.vi"("Numeric Array"=w418, "Name"=w409) -> ()  [unwired: 9 in, 1 out]
          n137 = call <vilib>:"WPI_RobotDriveDelayAndUpdateSafety.vi"("Delay (s)"=1.0, "RobotDriveDevRef"=w408) -> ("RobotDriveDevRef 2"=w407:T5)  [unwired: 8 in, 1 out]
        }
        frame #1 {
          # "Turn left 45 deg"
          n138 = while {
            shift-right: [w446] -> w427
            shift-left: w428 -> [w447]
            shift-right: [w443] -> w425
            shift-left: w426 -> [w444]
            tunnel: w424 -> [w437]
            tunnel: [w437] -> w423
            stop <- w431 stop-if-true
            w435 = -45.0 ("setpoint")
            n139 = call <vilib>:"ADI_IMU_ADIS16448_Get Angles.vi"("ADI IMU Interrupt DevRef"=w444) -> ("IMU Angles Out"=w445:T23, "ADI IMU Interrupt DevRef Out"=w443:T15)  [unwired: 7 in, 2 out]
            n140 = Unbundle By Name(w445) -> ("Z Angle"=w436:dbl)
            n141 = call-poly <vilib>:"PID.vi"("output range"=cluster{"output high":dbl, "output low":dbl} {"output high"=0.6, "output low"=-0.6}, "PID gains"=T22 {"proportional gain (Kc)"=1.0, "integral time (Ti, min)"=0.0, "derivative time (Td, min)"=0.0}, "process variable"=w436, "setpoint"=w435) -> ("output"=w440:dbl)  [unwired: 6 in, 1 out]
            n142 = Subtract(x=w436, y=w435) -> (x-y=w434:dbl)
            n143 = call-poly <vilib>:"WPI_RobotDriveArcadeDrive.vi"("Y axis value"=0.0, "X axis value"=w440, "RobotDriveDevRef"=w447) -> ("Motor Values"=w438:dbl[], "RobotDriveDevRef"=w446:T5)  [unwired: 6 in, 1 out]
            n144 = Absolute Value(x=w434) -> (abs(x)=w433:dbl)
            n145 = Wait (ms)(milliseconds to wait=u32 50) -> ()  [unwired: 1 out]
            n146 = Less?(x=w433, y=3.0) -> (x < y?=w431:bool)
            n147 = call-poly <vilib>:"NT Write Value.vi"("Numeric Array"=w438, "Name"=w437) -> ()  [unwired: 9 in, 1 out]
          }
        }
        frame #2 {
          # "stand still"
          n148 = call-poly <vilib>:"WPI_RobotDriveArcadeDrive.vi"("Y axis value"=0.0 ("X axis value"), "X axis value"=0.0, "RobotDriveDevRef"=w450) -> ("Motor Values"=w454:dbl[], "RobotDriveDevRef"=w449:T5)  [unwired: 1 in, 6 out]
          n149 = call-poly <vilib>:"NT Write Value.vi"("Numeric Array"=w454, "Name"=w451) -> ()  [unwired: 9 in, 1 out]
        }
        frame #3 {
          n150 = Tick Count (ms)() -> (millisecond timer value=w465:u32)
          n151 = while {
            tunnel: w466 -> [w493]
            tunnel: w465 -> [w491]
            tunnel: w464 -> [w480]
            tunnel: w463 -> [w485]
            tunnel: [w484] -> w462
            tunnel: [w480] -> w461
            tunnel: 7.0 ("setpoint") -> [w475]
            tunnel: w459 -> [w474]
            stop <- w477 continue-if-true
            w483 = u32 50 ("milliseconds to wait")
            # "Drive straight until close to wall, 4s timeout"
            n152 = call <vilib>:"ADI_IMU_ADIS16448_Get Angles.vi"("ADI IMU Interrupt DevRef"=w474) -> ("IMU Angles Out"=w469:T23)  [unwired: 7 in, 3 out]
            n153 = call-poly <vilib>:"WPI_UltrasonicGetRange.vi"("SonarMB1010AnalogDevRef"=w493) -> ("Distance"=w487:dbl)  [unwired: 8 in, 2 out]
            n154 = Wait (ms)(milliseconds to wait=w483) -> ()  [unwired: 1 out]
            n155 = Unbundle By Name(w469) -> ("Z Angle"=w468:dbl)
            n156 = Divide(x=w483, y=u32 1000) -> (x/y=w481:dbl)
            n157 = call-poly <vilib>:"PID.vi"("output range"=cluster{"output high":dbl, "output low":dbl} {"output high"=-0.7, "output low"=0.0}, "dt (s)"=w481, "PID gains"=T22 {"proportional gain (Kc)"=0.03, "integral time (Ti, min)"=0.0, "derivative time (Td, min)"=0.0003}, "process variable"=w487, "setpoint"=w475) -> ("output"=w467:dbl)  [unwired: 5 in, 1 out]
            n158 = Add(x=w491, y=u32 3000) -> (x+y=w479:u32)
            n159 = call-poly <vilib>:"PID.vi"("output range"=cluster{"output high":dbl, "output low":dbl} {"output high"=0.5, "output low"=-0.5}, "PID gains"=T22 {"proportional gain (Kc)"=0.1, "integral time (Ti, min)"=0.0, "derivative time (Td, min)"=0.0}, "process variable"=w468, "setpoint"=0.0) -> ("output"=w471:dbl)  [unwired: 6 in, 1 out]
            n160 = Tick Count (ms)() -> (millisecond timer value=w478:u32)
            n161 = Greater?(x=w479, y=w478) -> (0:w476:bool)
            n162 = call-poly <vilib>:"WPI_RobotDriveArcadeDrive.vi"("Y axis value"=w467, "X axis value"=w471, "RobotDriveDevRef"=w485) -> ("Motor Values"=w486:dbl[], "RobotDriveDevRef"=w484:T5)  [unwired: 6 in, 1 out]
            n163 = Greater?(x=w487, y=w475) -> (0:w492:bool)
            n164 = And(x=w476, y=w492) -> (x .and. y?=w477:bool)
            n165 = call-poly <vilib>:"NT Write Value.vi"("Numeric Array"=w486, "Name"=w480) -> ()  [unwired: 9 in, 1 out]
          }
        }
        frame #4 {
          # "Stop"
          n166 = call-poly <vilib>:"WPI_RobotDriveArcadeDrive.vi"("Y axis value"=0.0, "X axis value"=0.0, "RobotDriveDevRef"=w501) -> ("Motor Values"=w500:dbl[], "RobotDriveDevRef"=w497:T5)  [unwired: 6 in, 1 out]
          n167 = call-poly <vilib>:"NT Write Value.vi"("Numeric Array"=w500, "Name"=w494) -> ()  [unwired: 9 in, 1 out]
          n168 = call <vilib>:"WPI_RobotDriveDelayAndUpdateSafety.vi"("Delay (s)"=1.0, "RobotDriveDevRef"=w497) -> ("RobotDriveDevRef 2"=w502:T5)  [unwired: 8 in, 1 out]
        }
      }
      n169 = call <vilib>:"WPI_RobotDriveSafetyConfig.vi"("mode"=WPI_SafetyOutputConfigMenu."Enable", "RobotDriveDevRef"=w378) -> ()  [unwired: 8 in, 2 out]
    }
    frame "Right Gear" {
      n170 = call <vilib>:"ADI_IMU_ADIS16448_Reset.vi"("ADI IMU Interrupt DevRef"=w542) -> ("ADI IMU Interrupt DevRef Out"=w540:T15)  [unwired: 9 in, 1 out]
      n171 = call <vilib>:"WPI_RobotDriveSafetyConfig.vi"("mode"=WPI_SafetyOutputConfigMenu."Disable", "RobotDriveDevRef"=w537) -> ("RobotDriveDevRef"=w536:T5)  [unwired: 8 in, 1 out]
      n172 = flat-sequence {
        tunnel: w538 -> [w555]
        tunnel: w536 -> [w545]
        tunnel: w539 -> [w544]
        tunnel: w540 -> [w556]
        tunnel: w541 -> [w557]
        tunnel: [w557] -> w507
        tunnel: [w556] -> w506
        tunnel: [w544] -> w505
        tunnel: [w543] -> w504
        tunnel: [w555] -> w503
        tunnel: [w565] -> w512
        tunnel: [w560] -> w511
        tunnel: [w558] -> w510
        tunnel: [w562] -> w509
        tunnel: [w564] -> w508
        tunnel: w507 -> [w565]
        tunnel: w506 -> [w561]
        tunnel: w505 -> [w559]
        tunnel: w504 -> [w563]
        tunnel: w503 -> [w564]
        tunnel: [w592] -> w517
        tunnel: [w591] -> w516
        tunnel: [w586] -> w515
        tunnel: [w584] -> w514
        tunnel: [w590] -> w513
        tunnel: w512 -> [w592]
        tunnel: w511 -> [w591]
        tunnel: w510 -> [w586]
        tunnel: w509 -> [w585]
        tunnel: w508 -> [w590]
        tunnel: [w597] -> w532
        tunnel: [w596] -> w531
        tunnel: [w593] -> w528
        tunnel: w517 -> [w601]
        tunnel: w516 -> [w594]
        tunnel: w515 -> [w599]
        tunnel: w514 -> [w598]
        tunnel: w513 -> [w593]
        tunnel: w532 -> [w637]
        tunnel: w531 -> [w633]
        tunnel: [w630] -> w530
        tunnel: [w633] -> w529
        tunnel: w528 -> [w632]
        tunnel: [w632] -> w527
        tunnel: w530 -> [w643]
        tunnel: w529 -> [w642]
        tunnel: w527 -> [w641]
        tunnel: [w643] -> w526
        tunnel: [w642] -> w525
        tunnel: [w640] -> w524
        tunnel: w526 -> [w646]
        tunnel: w525 -> [w644]
        tunnel: w524 -> [w652]
        tunnel: [w645] -> w523
        tunnel: [w644] -> w522
        tunnel: [w652] -> w521
        tunnel: w523 -> [w655]
        tunnel: w522 -> [w653]
        tunnel: w521 -> [w661]
        tunnel: [w654] -> w520
        tunnel: [w653] -> w519
        tunnel: [w661] -> w518
        tunnel: [w664] -> _
        tunnel: [w665] -> w534
        tunnel: w520 -> [w665]
        tunnel: w519 -> [w664]
        tunnel: w518 -> [w662]
        frame #0 {
          # "stand still"
          # "Drive straight (timed)"
          n173 = call-poly <vilib>:"WPI_RobotDriveArcadeDrive.vi"("Y axis value"=-0.85 ("X axis value"), "X axis value"=0.0, "RobotDriveDevRef"=w545) -> ("Motor Values"=w554:dbl[], "RobotDriveDevRef"=w548:T5)  [unwired: 1 in, 6 out]
          n174 = call-poly <vilib>:"NT Write Value.vi"("Numeric Array"=w554, "Name"=w544) -> ()  [unwired: 9 in, 1 out]
          n175 = call <vilib>:"WPI_RobotDriveDelayAndUpdateSafety.vi"("Delay (s)"=2.0, "RobotDriveDevRef"=w548) -> ("RobotDriveDevRef 2"=w546:T5)  [unwired: 8 in, 1 out]
          n176 = call-poly <vilib>:"WPI_RobotDriveArcadeDrive.vi"("Y axis value"=0.0 ("X axis value"), "X axis value"=0.0, "RobotDriveDevRef"=w546) -> ("Motor Values"=w553:dbl[], "RobotDriveDevRef"=w543:T5)  [unwired: 1 in, 6 out]
          n177 = call-poly <vilib>:"NT Write Value.vi"("Numeric Array"=w553, "Name"=w544) -> ()  [unwired: 9 in, 1 out]
        }
        frame #1 {
          # "Turn left 45 deg"
          n178 = while {
            shift-right: [w581] -> w562
            shift-left: w563 -> [w582]
            shift-right: [w578] -> w560
            shift-left: w561 -> [w579]
            tunnel: w559 -> [w572]
            tunnel: [w572] -> w558
            stop <- w566 stop-if-true
            w570 = 45.0 ("setpoint")
            n179 = call <vilib>:"ADI_IMU_ADIS16448_Get Angles.vi"("ADI IMU Interrupt DevRef"=w579) -> ("IMU Angles Out"=w580:T23, "ADI IMU Interrupt DevRef Out"=w578:T15)  [unwired: 7 in, 2 out]
            n180 = Unbundle By Name(w580) -> ("Z Angle"=w571:dbl)
            n181 = call-poly <vilib>:"PID.vi"("output range"=cluster{"output high":dbl, "output low":dbl} {"output high"=0.3, "output low"=-0.3}, "PID gains"=T22 {"proportional gain (Kc)"=0.1, "integral time (Ti, min)"=0.0, "derivative time (Td, min)"=0.0}, "process variable"=w571, "setpoint"=w570) -> ("output"=w575:dbl)  [unwired: 6 in, 1 out]
            n182 = Subtract(x=w571, y=w570) -> (x-y=w569:dbl)
            n183 = call-poly <vilib>:"WPI_RobotDriveArcadeDrive.vi"("Y axis value"=0.0, "X axis value"=w575, "RobotDriveDevRef"=w582) -> ("Motor Values"=w573:dbl[], "RobotDriveDevRef"=w581:T5)  [unwired: 6 in, 1 out]
            n184 = Absolute Value(x=w569) -> (abs(x)=w568:dbl)
            n185 = Wait (ms)(milliseconds to wait=u32 50) -> ()  [unwired: 1 out]
            n186 = Less?(x=w568, y=3.0) -> (x < y?=w566:bool)
            n187 = call-poly <vilib>:"NT Write Value.vi"("Numeric Array"=w573, "Name"=w572) -> ()  [unwired: 9 in, 1 out]
          }
        }
        frame #2 {
          # "stand still"
          n188 = call-poly <vilib>:"WPI_RobotDriveArcadeDrive.vi"("Y axis value"=0.0 ("X axis value"), "X axis value"=0.0, "RobotDriveDevRef"=w585) -> ("Motor Values"=w589:dbl[], "RobotDriveDevRef"=w584:T5)  [unwired: 1 in, 6 out]
          n189 = call-poly <vilib>:"NT Write Value.vi"("Numeric Array"=w589, "Name"=w586) -> ()  [unwired: 9 in, 1 out]
        }
        frame #3 {
          n190 = Tick Count (ms)() -> (millisecond timer value=w600:u32)
          n191 = while {
            tunnel: w601 -> [w628]
            tunnel: w600 -> [w626]
            tunnel: w599 -> [w615]
            tunnel: w598 -> [w620]
            tunnel: [w619] -> w597
            tunnel: [w615] -> w596
            tunnel: 7.0 ("setpoint") -> [w610]
            tunnel: w594 -> [w609]
            stop <- w612 continue-if-true
            w618 = u32 50 ("milliseconds to wait")
            # "Drive straight until close to wall, 4s timeout"
            n192 = call <vilib>:"ADI_IMU_ADIS16448_Get Angles.vi"("ADI IMU Interrupt DevRef"=w609) -> ("IMU Angles Out"=w604:T23)  [unwired: 7 in, 3 out]
            n193 = call-poly <vilib>:"WPI_UltrasonicGetRange.vi"("SonarMB1010AnalogDevRef"=w628) -> ("Distance"=w622:dbl)  [unwired: 8 in, 2 out]
            n194 = Wait (ms)(milliseconds to wait=w618) -> ()  [unwired: 1 out]
            n195 = Unbundle By Name(w604) -> ("Z Angle"=w603:dbl)
            n196 = Divide(x=w618, y=u32 1000) -> (x/y=w616:dbl)
            n197 = call-poly <vilib>:"PID.vi"("output range"=cluster{"output high":dbl, "output low":dbl} {"output high"=-0.7, "output low"=0.0}, "dt (s)"=w616, "PID gains"=T22 {"proportional gain (Kc)"=0.03, "integral time (Ti, min)"=0.0, "derivative time (Td, min)"=0.0003}, "process variable"=w622, "setpoint"=w610) -> ("output"=w602:dbl)  [unwired: 5 in, 1 out]
            n198 = Add(x=w626, y=u32 4000) -> (x+y=w614:u32)
            n199 = call-poly <vilib>:"PID.vi"("output range"=cluster{"output high":dbl, "output low":dbl} {"output high"=0.5, "output low"=-0.5}, "PID gains"=T22 {"proportional gain (Kc)"=0.1, "integral time (Ti, min)"=0.0, "derivative time (Td, min)"=0.0}, "process variable"=w603, "setpoint"=0.0) -> ("output"=w606:dbl)  [unwired: 6 in, 1 out]
            n200 = Tick Count (ms)() -> (millisecond timer value=w613:u32)
            n201 = Greater?(x=w614, y=w613) -> (0:w611:bool)
            n202 = call-poly <vilib>:"WPI_RobotDriveArcadeDrive.vi"("Y axis value"=w602, "X axis value"=w606, "RobotDriveDevRef"=w620) -> ("Motor Values"=w621:dbl[], "RobotDriveDevRef"=w619:T5)  [unwired: 6 in, 1 out]
            n203 = Greater?(x=w622, y=w610) -> (0:w627:bool)
            n204 = And(x=w611, y=w627) -> (x .and. y?=w612:bool)
            n205 = call-poly <vilib>:"NT Write Value.vi"("Numeric Array"=w621, "Name"=w615) -> ()  [unwired: 9 in, 1 out]
          }
        }
        frame #4 {
          # "Stop"
          n206 = call-poly <vilib>:"WPI_RobotDriveArcadeDrive.vi"("Y axis value"=0.0, "X axis value"=0.0, "RobotDriveDevRef"=w637) -> ("Motor Values"=w636:dbl[], "RobotDriveDevRef"=w631:T5)  [unwired: 6 in, 1 out]
          n207 = call-poly <vilib>:"NT Write Value.vi"("Numeric Array"=w636, "Name"=w633) -> ()  [unwired: 9 in, 1 out]
          n208 = call <vilib>:"WPI_RobotDriveDelayAndUpdateSafety.vi"("Delay (s)"=1.0, "RobotDriveDevRef"=w631) -> ("RobotDriveDevRef 2"=w630:T5)  [unwired: 8 in, 1 out]
        }
        frame #5 {
          n209 = call-poly <vilib>:"WPI_SolenoidSet.vi"("Value"=WPI_SolenoidValue."Forward", "SolenoidDevRef"=w641) -> ("SolenoidDevRef"=w640:T13)  [unwired: 8 in, 1 out]
          n210 = Wait (ms)(milliseconds to wait=u32 1000) -> ()  [unwired: 1 out]
        }
        frame #6 {
          n211 = call-poly <vilib>:"WPI_RobotDriveArcadeDrive.vi"("Y axis value"=0.7 ("X axis value"), "X axis value"=0.0, "RobotDriveDevRef"=w646) -> ("Motor Values"=w651:dbl[], "RobotDriveDevRef"=w648:T5)  [unwired: 1 in, 6 out]
          n212 = call <vilib>:"WPI_RobotDriveDelayAndUpdateSafety.vi"("Delay (s)"=1.0, "RobotDriveDevRef"=w648) -> ("RobotDriveDevRef 2"=w645:T5)  [unwired: 8 in, 1 out]
          n213 = call-poly <vilib>:"NT Write Value.vi"("Numeric Array"=w651, "Name"=w644) -> ()  [unwired: 9 in, 1 out]
        }
        frame #7 {
          n214 = call-poly <vilib>:"WPI_RobotDriveArcadeDrive.vi"("Y axis value"=0.0 ("X axis value"), "X axis value"=0.0, "RobotDriveDevRef"=w655) -> ("Motor Values"=w660:dbl[], "RobotDriveDevRef"=w658:T5)  [unwired: 1 in, 6 out]
          n215 = call-poly <vilib>:"NT Write Value.vi"("Numeric Array"=w660, "Name"=w653) -> ()  [unwired: 9 in, 1 out]
          n216 = call <vilib>:"WPI_RobotDriveDelayAndUpdateSafety.vi"("Delay (s)"=1.0, "RobotDriveDevRef"=w658) -> ("RobotDriveDevRef 2"=w654:T5)  [unwired: 8 in, 1 out]
        }
        frame #8 {
          n217 = call-poly <vilib>:"WPI_SolenoidSet.vi"("Value"=WPI_SolenoidValue."Reverse", "SolenoidDevRef"=w662) -> ()  [unwired: 8 in, 2 out]
        }
      }
      n218 = call <vilib>:"WPI_RobotDriveSafetyConfig.vi"("mode"=WPI_SafetyOutputConfigMenu."Enable", "RobotDriveDevRef"=w534) -> ()  [unwired: 8 in, 2 out]
    }
    frame "Right Gear no drop gear" {
      n219 = call <vilib>:"ADI_IMU_ADIS16448_Reset.vi"("ADI IMU Interrupt DevRef"=w693) -> ("ADI IMU Interrupt DevRef Out"=w691:T15)  [unwired: 9 in, 1 out]
      n220 = call <vilib>:"WPI_RobotDriveSafetyConfig.vi"("mode"=WPI_SafetyOutputConfigMenu."Disable", "RobotDriveDevRef"=w688) -> ("RobotDriveDevRef"=w687:T5)  [unwired: 8 in, 1 out]
      n221 = flat-sequence {
        tunnel: w689 -> [w708]
        tunnel: w687 -> [w698]
        tunnel: w690 -> [w697]
        tunnel: w691 -> [w709]
        tunnel: w692 -> [w710]
        tunnel: [w710] -> w671
        tunnel: [w709] -> w670
        tunnel: [w697] -> w669
        tunnel: [w695] -> w668
        tunnel: [w708] -> w667
        tunnel: [w718] -> w676
        tunnel: [w713] -> w675
        tunnel: [w711] -> w674
        tunnel: [w715] -> w673
        tunnel: [w717] -> w672
        tunnel: w671 -> [w718]
        tunnel: w670 -> [w714]
        tunnel: w669 -> [w712]
        tunnel: w668 -> [w716]
        tunnel: w667 -> [w717]
        tunnel: [w745] -> w681
        tunnel: [w744] -> w680
        tunnel: [w739] -> w679
        tunnel: [w737] -> w678
        tunnel: [w743] -> w677
        tunnel: w676 -> [w745]
        tunnel: w675 -> [w744]
        tunnel: w674 -> [w739]
        tunnel: w673 -> [w738]
        tunnel: w672 -> [w743]
        tunnel: [w750] -> w684
        tunnel: [w749] -> w683
        tunnel: [w746] -> w682
        tunnel: w681 -> [w754]
        tunnel: w680 -> [w747]
        tunnel: w679 -> [w752]
        tunnel: w678 -> [w751]
        tunnel: w677 -> [w746]
        tunnel: [w790] -> w666
        tunnel: w682 -> [w782]
        tunnel: w683 -> [w783]
        tunnel: w684 -> [w789]
        tunnel: [w783] -> _
        tunnel: [w782] -> _
        frame #0 {
          # "stand still"
          # "Drive straight (timed)"
          n222 = call-poly <vilib>:"WPI_RobotDriveArcadeDrive.vi"("Y axis value"=-0.7 ("X axis value"), "X axis value"=0.0, "RobotDriveDevRef"=w698) -> ("Motor Values"=w707:dbl[], "RobotDriveDevRef"=w701:T5)  [unwired: 1 in, 6 out]
          n223 = call-poly <vilib>:"NT Write Value.vi"("Numeric Array"=w707, "Name"=w697) -> ()  [unwired: 9 in, 1 out]
          n224 = call <vilib>:"WPI_RobotDriveDelayAndUpdateSafety.vi"("Delay (s)"=2.0, "RobotDriveDevRef"=w701) -> ("RobotDriveDevRef 2"=w699:T5)  [unwired: 8 in, 1 out]
          n225 = call-poly <vilib>:"WPI_RobotDriveArcadeDrive.vi"("Y axis value"=0.0 ("X axis value"), "X axis value"=0.0, "RobotDriveDevRef"=w699) -> ("Motor Values"=w706:dbl[], "RobotDriveDevRef"=w696:T5)  [unwired: 1 in, 6 out]
          n226 = call-poly <vilib>:"NT Write Value.vi"("Numeric Array"=w706, "Name"=w697) -> ()  [unwired: 9 in, 1 out]
          n227 = call <vilib>:"WPI_RobotDriveDelayAndUpdateSafety.vi"("Delay (s)"=1.0, "RobotDriveDevRef"=w696) -> ("RobotDriveDevRef 2"=w695:T5)  [unwired: 8 in, 1 out]
        }
        frame #1 {
          # "Turn left 45 deg"
          n228 = while {
            shift-right: [w734] -> w715
            shift-left: w716 -> [w735]
            shift-right: [w731] -> w713
            shift-left: w714 -> [w732]
            tunnel: w712 -> [w725]
            tunnel: [w725] -> w711
            stop <- w719 stop-if-true
            w723 = 45.0 ("setpoint")
            n229 = call <vilib>:"ADI_IMU_ADIS16448_Get Angles.vi"("ADI IMU Interrupt DevRef"=w732) -> ("IMU Angles Out"=w733:T23, "ADI IMU Interrupt DevRef Out"=w731:T15)  [unwired: 7 in, 2 out]
            n230 = Unbundle By Name(w733) -> ("Z Angle"=w724:dbl)
            n231 = call-poly <vilib>:"PID.vi"("output range"=cluster{"output high":dbl, "output low":dbl} {"output high"=0.6, "output low"=-0.6}, "PID gains"=T22 {"proportional gain (Kc)"=1.0, "integral time (Ti, min)"=0.0, "derivative time (Td, min)"=0.0}, "process variable"=w724, "setpoint"=w723) -> ("output"=w728:dbl)  [unwired: 6 in, 1 out]
            n232 = Subtract(x=w724, y=w723) -> (x-y=w722:dbl)
            n233 = call-poly <vilib>:"WPI_RobotDriveArcadeDrive.vi"("Y axis value"=0.0, "X axis value"=w728, "RobotDriveDevRef"=w735) -> ("Motor Values"=w726:dbl[], "RobotDriveDevRef"=w734:T5)  [unwired: 6 in, 1 out]
            n234 = Absolute Value(x=w722) -> (abs(x)=w721:dbl)
            n235 = Wait (ms)(milliseconds to wait=u32 50) -> ()  [unwired: 1 out]
            n236 = Less?(x=w721, y=2.0) -> (x < y?=w719:bool)
            n237 = call-poly <vilib>:"NT Write Value.vi"("Numeric Array"=w726, "Name"=w725) -> ()  [unwired: 9 in, 1 out]
          }
        }
        frame #2 {
          # "stand still"
          n238 = call-poly <vilib>:"WPI_RobotDriveArcadeDrive.vi"("Y axis value"=0.0 ("X axis value"), "X axis value"=0.0, "RobotDriveDevRef"=w738) -> ("Motor Values"=w742:dbl[], "RobotDriveDevRef"=w737:T5)  [unwired: 1 in, 6 out]
          n239 = call-poly <vilib>:"NT Write Value.vi"("Numeric Array"=w742, "Name"=w739) -> ()  [unwired: 9 in, 1 out]
        }
        frame #3 {
          n240 = Tick Count (ms)() -> (millisecond timer value=w753:u32)
          n241 = while {
            tunnel: w754 -> [w781]
            tunnel: w753 -> [w779]
            tunnel: w752 -> [w768]
            tunnel: w751 -> [w773]
            tunnel: [w772] -> w750
            tunnel: [w768] -> w749
            tunnel: 7.0 ("setpoint") -> [w763]
            tunnel: w747 -> [w762]
            stop <- w765 continue-if-true
            w771 = u32 50 ("milliseconds to wait")
            # "Drive straight until close to wall, 4s timeout"
            n242 = call <vilib>:"ADI_IMU_ADIS16448_Get Angles.vi"("ADI IMU Interrupt DevRef"=w762) -> ("IMU Angles Out"=w757:T23)  [unwired: 7 in, 3 out]
            n243 = call-poly <vilib>:"WPI_UltrasonicGetRange.vi"("SonarMB1010AnalogDevRef"=w781) -> ("Distance"=w775:dbl)  [unwired: 8 in, 2 out]
            n244 = Wait (ms)(milliseconds to wait=w771) -> ()  [unwired: 1 out]
            n245 = Unbundle By Name(w757) -> ("Z Angle"=w756:dbl)
            n246 = Divide(x=w771, y=u32 1000) -> (x/y=w769:dbl)
            n247 = call-poly <vilib>:"PID.vi"("output range"=cluster{"output high":dbl, "output low":dbl} {"output high"=-0.7, "output low"=0.0}, "dt (s)"=w769, "PID gains"=T22 {"proportional gain (Kc)"=1.0, "integral time (Ti, min)"=0.01, "derivative time (Td, min)"=0.0001}, "process variable"=w775, "setpoint"=w763) -> ("output"=w755:dbl)  [unwired: 5 in, 1 out]
            n248 = Add(x=w779, y=u32 4000) -> (x+y=w767:u32)
            n249 = call-poly <vilib>:"PID.vi"("output range"=cluster{"output high":dbl, "output low":dbl} {"output high"=0.5, "output low"=-0.5}, "PID gains"=T22 {"proportional gain (Kc)"=0.1, "integral time (Ti, min)"=0.0, "derivative time (Td, min)"=0.0}, "process variable"=w756, "setpoint"=45.0) -> ("output"=w759:dbl)  [unwired: 6 in, 1 out]
            n250 = Tick Count (ms)() -> (millisecond timer value=w766:u32)
            n251 = Greater?(x=w767, y=w766) -> (0:w764:bool)
            n252 = call-poly <vilib>:"WPI_RobotDriveArcadeDrive.vi"("Y axis value"=w755, "X axis value"=w759, "RobotDriveDevRef"=w773) -> ("Motor Values"=w774:dbl[], "RobotDriveDevRef"=w772:T5)  [unwired: 6 in, 1 out]
            n253 = Greater?(x=w775, y=w763) -> (0:w780:bool)
            n254 = And(x=w764, y=w780) -> (x .and. y?=w765:bool)
            n255 = call-poly <vilib>:"NT Write Value.vi"("Numeric Array"=w774, "Name"=w768) -> ()  [unwired: 9 in, 1 out]
          }
        }
        frame #4 {
          # "Stop"
          n256 = call-poly <vilib>:"WPI_RobotDriveArcadeDrive.vi"("Y axis value"=0.0, "X axis value"=0.0, "RobotDriveDevRef"=w789) -> ("Motor Values"=w788:dbl[], "RobotDriveDevRef"=w785:T5)  [unwired: 6 in, 1 out]
          n257 = call-poly <vilib>:"NT Write Value.vi"("Numeric Array"=w788, "Name"=w783) -> ()  [unwired: 9 in, 1 out]
          n258 = call <vilib>:"WPI_RobotDriveDelayAndUpdateSafety.vi"("Delay (s)"=1.0, "RobotDriveDevRef"=w785) -> ("RobotDriveDevRef 2"=w790:T5)  [unwired: 8 in, 1 out]
        }
      }
      n259 = call <vilib>:"WPI_RobotDriveSafetyConfig.vi"("mode"=WPI_SafetyOutputConfigMenu."Enable", "RobotDriveDevRef"=w666) -> ()  [unwired: 8 in, 2 out]
    }
  }
  n260 = while {
    stop <- FALSE stop-if-true
    n261 = call <vilib>:"WPI_DriverStationReport Robot Code State.vi"("Autonomous"=TRUE) -> ()  [unwired: 10 in, 1 out]
    n262 = Wait (ms)(milliseconds to wait=u32 20) -> ()  [unwired: 1 out]
  }
